vi "Queue.vi"(0 "Element_In":dbl, 9 "Operation":T1=enum."Enqueue", 11 "Error_In":errorcluster) -> (3 "Overflow":bool, 4 "Element_Out":dbl, 6 "Sum":dbl, 14 "Underflow":bool, 15 "Error_Out":errorcluster)   [LabVIEW 2023]
doc: "This is a LV2, Which has array as its storage unit. hence can be used as queue. it is provided with the pins as follows\nElement_in - Data to be Enqueued\nElement_out - Data Dequeued\nSum - Provides the total sum of elelments in the queue\noverflow and underflow - flags that turns on when overflow and underflow conditions accours.\nError_in and Error_out where given for Error handling"
uses:
  Type_Def/Operation_Queue.ctl
  Type_Def/Queue_and_Pointer.ctl
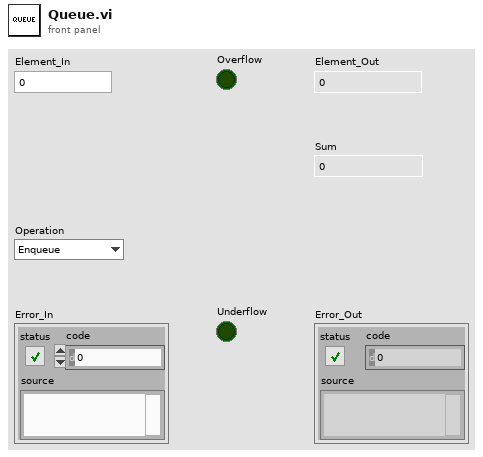
[diagram p1: front panel]
types:
  T1 = typedef "Operation_Queue.ctl" = enum16{"Initialize", "Enqueue", "Dequeue", "Sum"}
  T2 = typedef "Queue_and_Pointer.ctl" = cluster{"Head_Pointer":i64, "Dimension_Size (10)":i64, "Queue":dbl[]}
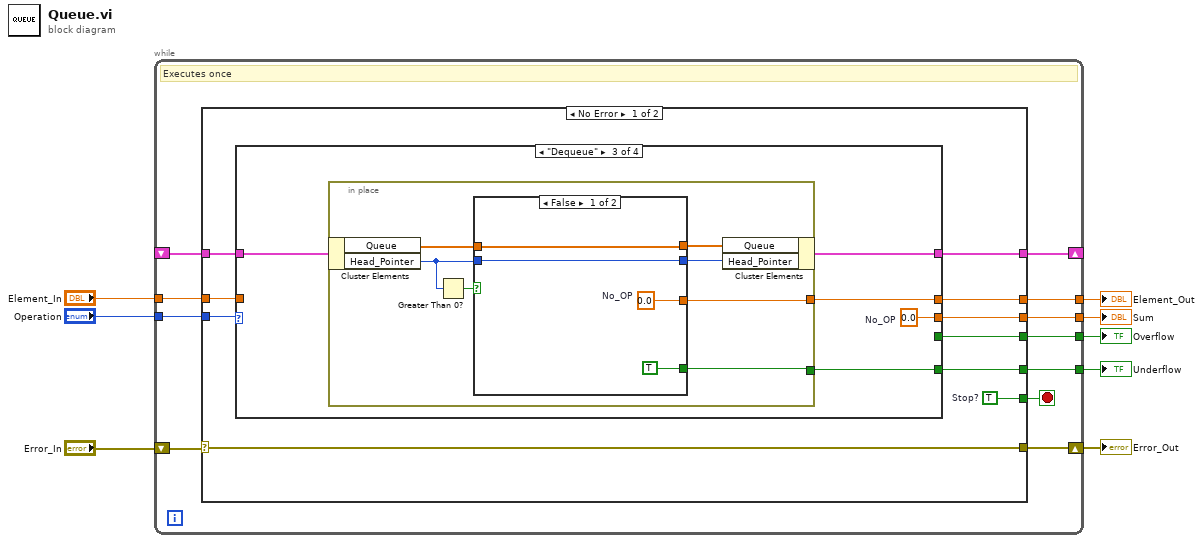
[diagram p0: block diagram]
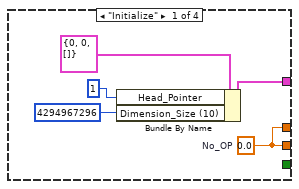
[diagram p2: hidden frame]
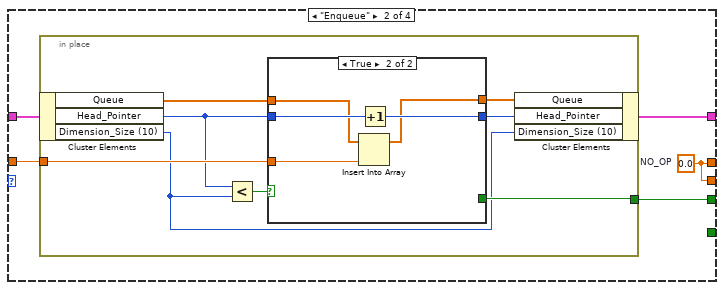
[diagram p3: hidden frame]
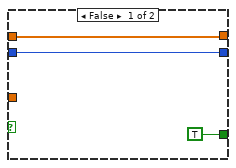
[diagram p4: hidden frame]
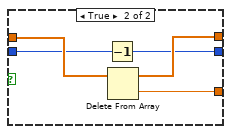
[diagram p5: hidden frame]
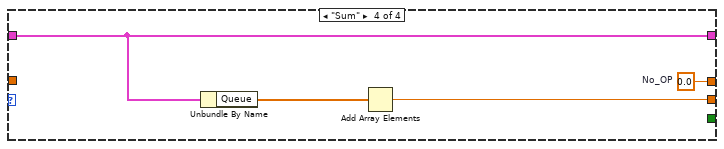
[diagram p6: hidden frame]
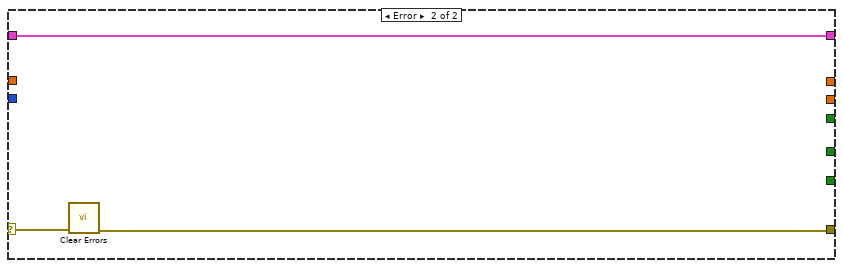
[diagram p7: hidden frame]
diagram:
  n1 = while {
    tunnel: [w19] -> w8
    tunnel: [w18] -> w7
    tunnel: "Element_In" -> [w17]
    tunnel: "Operation" -> [w16]
    tunnel: [w14] -> w4
    tunnel: [w13] -> w3
    shift-right: [w12] -> _
    shift-left: _ -> [w11]
    shift-right: [w9] -> w1
    shift-left: "Error_In" -> [w10]
    stop <- w15 stop-if-true
    # "Executes once"
    n2 = case shown="No Error" w10 {
      selector: w10 -> [w20 w83]
      tunnel: [w29 _] -> w19
      tunnel: [w28 _] -> w18
      tunnel: w17 -> [w27 _]
      tunnel: w16 -> [w26 _]
      tunnel: [w25 _] -> w15
      tunnel: [w24 _] -> w14
      tunnel: [w23 _] -> w13
      tunnel: [w22 w82] -> w12
      tunnel: w11 -> [w21 w82]
      tunnel: [w20 w81] -> w9
      frame No Error {
        w25 = TRUE  # Stop?
        n3 = case shown="\"Dequeue\"" w26 {
          tunnel: w21 -> [_ w36 w56 w79]
          tunnel: w27 -> [_ w39 _ _]
          tunnel: [w30 w37 w60 w80] -> w29
          tunnel: [w30 w37 w59 w78] -> w28
          tunnel: [_ w38 _ _] -> w24
          tunnel: [_ _ w58 _] -> w23
          tunnel: [w33 w35 w57 w79] -> w22
          frame "Initialize" {
            w30 = 0.0  # No_OP
            n4 = Bundle By Name(cluster=T2 {"Head_Pointer"=0, "Dimension_Size (10)"=0, "Queue"=[]} ("Queue_and_Pointer"), "Head_Pointer"=i64 1 ("Dimension_Size (10)"), "Dimension_Size (10)"=i64 4294967296) -> (w33:T2)
          }
          frame "Enqueue" {
            w37 = 0.0  # NO_OP
            n5 = in-place "In Place Element Structure" {
              in-place-border: w39 -> [w47]
              in-place-border: [w45] -> w38
              n6 = in-place-cluster #1(w36) -> ("Queue"=w44:dbl[], "Head_Pointer"=w41:i64, "Dimension_Size (10)"=w40:i64)
              n7 = Less?(x=w41, y=w40) -> (x < y?=w46:bool)
              n8 = case shown="True" w46 {
                tunnel: w47 -> [_ w52]
                tunnel: w44 -> [w49 w51]
                tunnel: [w49 w53] -> w42
                tunnel: w41 -> [w50 w55]
                tunnel: [w50 w54] -> w43
                tunnel: [TRUE _] -> w45
                frame False {
                }
                frame True {
                  n9 = Insert Into Array(array=w51, new element=w52) -> (w53:dbl[])  [unwired: 1 in]
                  n10 = Increment(x=w55) -> (x+1=w54:i64)
                }
              }
              n11 = in-place-cluster #1("Queue"=w42, "Head_Pointer"=w43, "Dimension_Size (10)"=w40) -> (w35:T2)
            }
          }
          frame "Dequeue" {
            w59 = 0.0  # No_OP
            n12 = in-place "In Place Element Structure" {
              in-place-border: [w67] -> w60
              in-place-border: [w65] -> w58
              n13 = in-place-cluster #2(w56) -> ("Queue"=w62:dbl[], "Head_Pointer"=w63:i64)
              n14 = Greater Than 0?(x=w63) -> (x > 0?=w64:bool)
              n15 = case shown="False" w64 {
                tunnel: [w71 w75] -> w61
                tunnel: w62 -> [w71 w76]
                tunnel: [w69 w74] -> w67
                tunnel: w63 -> [w70 w73]
                tunnel: [w70 w72] -> w66
                tunnel: [TRUE _] -> w65
                frame False {
                  w69 = 0.0  # No_OP
                }
                frame True {
                  n16 = Decrement(x=w73) -> (x-1=w72:i64)
                  n17 = Delete From Array(array=w76) -> (deleted portion=w74:dbl, array with subset deleted=w75:dbl[])  [unwired: 2 in]
                }
              }
              n18 = in-place-cluster #2("Queue"=w61, "Head_Pointer"=w66) -> (w57:T2)
            }
          }
          frame "Sum" {
            w80 = 0.0  # No_OP
            n19 = Unbundle By Name(w79) -> ("Queue"=w77:dbl[])
            n20 = Add Array Elements(numeric array=w77) -> (sum=w78:dbl)
          }
        }
      }
      frame Error {
        n21 = call <vilib>:"Clear Errors.vi"("error in (no error)"=w83) -> ("error out"=w81:errorcluster)  [unwired: 5 in, 1 out]
      }
    }
  }
  "Error_Out" <- w1
  "Element_Out" <- w8
  "Sum" <- w7
  "Overflow" <- w4
  "Underflow" <- w3
